vi "OP600ZP_Assembly.vi"(8 "DCIR_MESURES":cluster{dbl, dbl, dbl, dbl, dbl, dbl, dbl, dbl}) -> (0 "ToBDD":T1, 1 "Out":string, 3 "PASS/FAIL":bool)   [LabVIEW 2020]
uses:
  OP600ZP_VGConf.vi
  VG/PackType.vi
  VG/IS30%.vi
  VG/DCIR@1C.vi
  VG/Ubatt.vi
panel:
  out "errout":errorcluster caption="error out"
  in  "errin":errorcluster caption="error out"
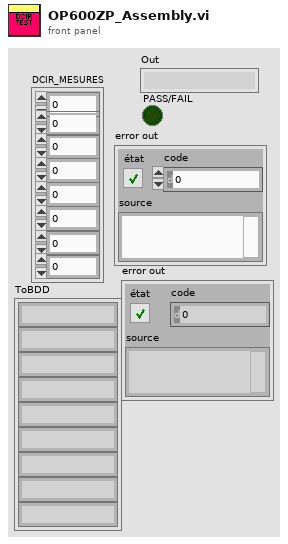
[diagram p1: front panel]
types:
  T1 = cluster{string, string, string, string, string, string, string, string, string}
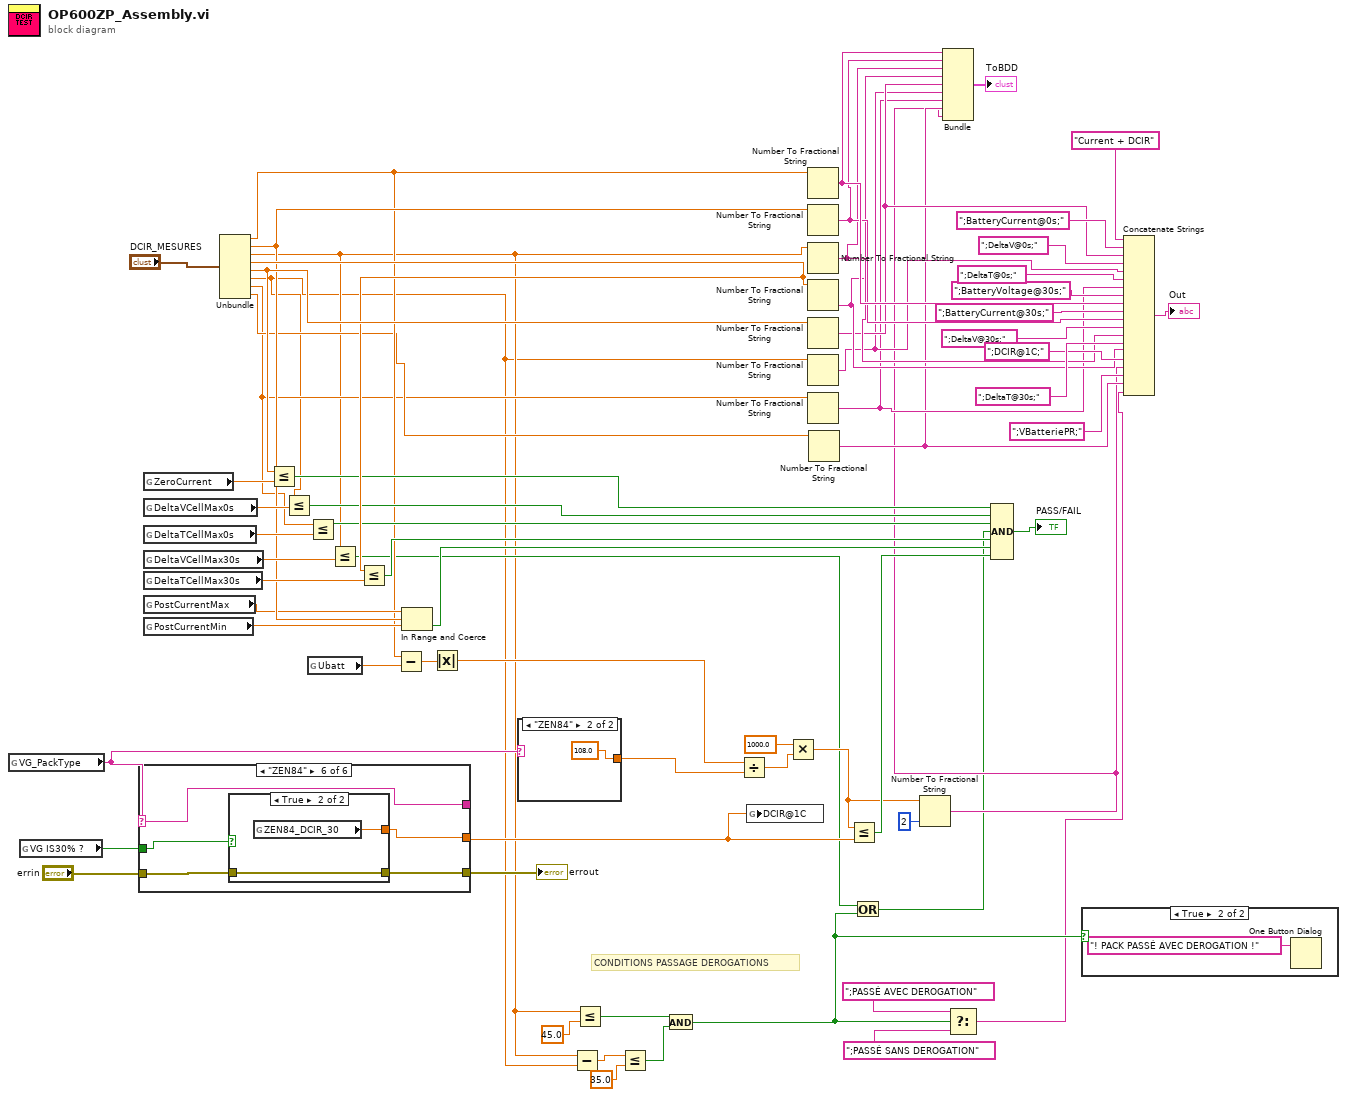
[diagram p0: block diagram]
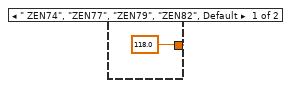
[diagram p3: hidden frame]
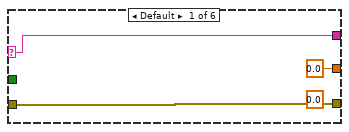
[diagram p4: hidden frame]
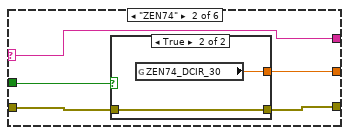
[diagram p5: hidden frame]
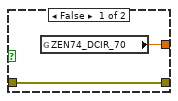
[diagram p6: hidden frame]
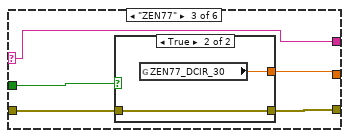
[diagram p7: hidden frame]
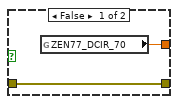
[diagram p8: hidden frame]
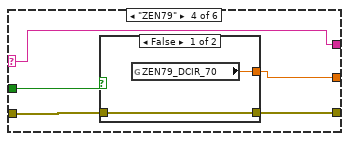
[diagram p9: hidden frame]
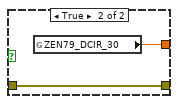
[diagram p10: hidden frame]
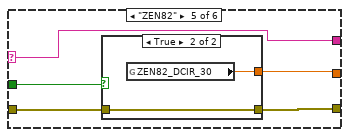
[diagram p11: hidden frame]
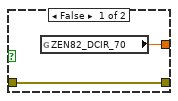
[diagram p12: hidden frame]
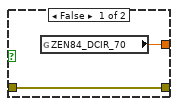
[diagram p13: hidden frame]
diagram:
  # "CONDITIONS PASSAGE DEROGATIONS"
  n1 = global read "PackType.vi" "VG_PackType"() -> (w36:string)
  n2 = global read "IS30%.vi" "VG IS30% ?"() -> (w42:bool)
  n3 = case shown="\"ZEN84\"" w36 {
    selector: w36 -> [w71 w74 w83 w92 w101 w110]
    tunnel: [0.0 ("ZEN84UbattMax30") w76 w85 w94 w103 w112] -> w32
    tunnel: w42 -> [_ w75 w84 w93 w102 w111]
    tunnel: [w71 w74 w83 w92 w101 w110] -> _
    tunnel: "errin" -> [w70 w73 w82 w91 w100 w109]
    tunnel: [w70 w72 w81 w90 w99 w108] -> w40
    frame Default {
      (unwired) 0.0 ("ZEN84UbattMin30")
    }
    frame "ZEN74" {
      n4 = case shown="True" w75 {
        tunnel: [w78 w80] -> w76
        tunnel: [w77 w79] -> w72
        tunnel: w73 -> [w77 w79]
        frame False {
          n5 = global read "OP600ZP_VGConf.vi" "ZEN74_DCIR_70"() -> (w78:dbl)
        }
        frame True {
          n6 = global read "OP600ZP_VGConf.vi" "ZEN74_DCIR_30"() -> (w80:dbl)
        }
      }
    }
    frame "ZEN77" {
      n7 = case shown="True" w84 {
        tunnel: [w87 w89] -> w85
        tunnel: w82 -> [w86 w88]
        tunnel: [w86 w88] -> w81
        frame False {
          n8 = global read "OP600ZP_VGConf.vi" "ZEN77_DCIR_70"() -> (w87:dbl)
        }
        frame True {
          n9 = global read "OP600ZP_VGConf.vi" "ZEN77_DCIR_30"() -> (w89:dbl)
        }
      }
    }
    frame "ZEN79" {
      n10 = case shown="False" w93 {
        tunnel: [w96 w98] -> w94
        tunnel: w91 -> [w95 w97]
        tunnel: [w95 w97] -> w90
        frame False {
          n11 = global read "OP600ZP_VGConf.vi" "ZEN79_DCIR_70"() -> (w96:dbl)
        }
        frame True {
          n12 = global read "OP600ZP_VGConf.vi" "ZEN79_DCIR_30"() -> (w98:dbl)
        }
      }
    }
    frame "ZEN82" {
      n13 = case shown="True" w102 {
        tunnel: [w105 w107] -> w103
        tunnel: w100 -> [w104 w106]
        tunnel: [w104 w106] -> w99
        frame False {
          n14 = global read "OP600ZP_VGConf.vi" "ZEN82_DCIR_70"() -> (w105:dbl)
        }
        frame True {
          n15 = global read "OP600ZP_VGConf.vi" "ZEN82_DCIR_30"() -> (w107:dbl)
        }
      }
    }
    frame "ZEN84" {
      n16 = case shown="True" w111 {
        tunnel: [w114 w116] -> w112
        tunnel: w109 -> [w113 w115]
        tunnel: [w113 w115] -> w108
        frame False {
          n17 = global read "OP600ZP_VGConf.vi" "ZEN84_DCIR_70"() -> (w114:dbl)
        }
        frame True {
          n18 = global read "OP600ZP_VGConf.vi" "ZEN84_DCIR_30"() -> (w116:dbl)
        }
      }
    }
  }
  "errout" <- w40
  n19 = global read "OP600ZP_VGConf.vi" "ZeroCurrent"() -> (w67:dbl)
  n20 = global read "OP600ZP_VGConf.vi" "DeltaVCellMax0s"() -> (w55:dbl)
  n21 = global read "OP600ZP_VGConf.vi" "DeltaTCellMax0s"() -> (w54:dbl)
  n22 = global read "OP600ZP_VGConf.vi" "DeltaVCellMax30s"() -> (w53:dbl)
  n23 = global read "OP600ZP_VGConf.vi" "DeltaTCellMax30s"() -> (w52:dbl)
  n24 = global read "OP600ZP_VGConf.vi" "PostCurrentMax"() -> (w49:dbl)
  n25 = global read "OP600ZP_VGConf.vi" "PostCurrentMin"() -> (w48:dbl)
  n26 = Unbundle("DCIR_MESURES") -> (w39:dbl, w50:dbl, w3:dbl, w51:dbl, w57:dbl, w2:dbl, w24:dbl, w26:dbl)
  n27 = Less Or Equal?(x=w57, y=w67) -> (x <= y?=w47:bool)
  n28 = Less Or Equal?(x=w2, y=w55) -> (x <= y?=w46:bool)
  n29 = Less Or Equal?(x=w24, y=w54) -> (x <= y?=w45:bool)
  n30 = global read "Ubatt.vi" "Ubatt"() -> (w38:dbl)
  n31 = Less Or Equal?(x=w3, y=w53) -> (x <= y?=w5:bool)
  n32 = Less Or Equal?(x=w51, y=w52) -> (x <= y?=w44:bool)
  n33 = Subtract(x=w39, y=w38) -> (x-y=w37:dbl)
  n34 = In Range and Coerce(upper limit=w49, x=w50, lower limit=w48) -> (In Range?=w43:bool)  [unwired: 1 out]
  n35 = Absolute Value(x=w37) -> (abs(x)=w35:dbl)
  n36 = case shown="\"ZEN84\"" w36 {
    tunnel: [118.0 108.0] -> w30
    frame " ZEN74", "ZEN77", "ZEN79", "ZEN82", Default {
    }
    frame "ZEN84" {
    }
  }
  n37 = Subtract(x=w3, y=w2) -> (x-y=w11:dbl)
  n38 = Less Or Equal?(x=w3, y=45.0) -> (x <= y?=w12:bool)
  n39 = Less Or Equal?(x=w11, y=35.0) -> (x <= y?=w9:bool)
  n40 = And(x=w12, y=w9) -> (x .and. y?=w6:bool)
  n41 = Divide(x=w35, y=w30) -> (x/y=w28:dbl)
  n42 = global write "DCIR@1C.vi" "DCIR@1C"(w32) -> ()
  n43 = Multiply(x=1000.0, y=w28) -> (x*y=w27:dbl)
  n44 = Number To Fractional String(number=w39) -> (F-format string=w23:string)  [unwired: 3 in]
  n45 = Number To Fractional String(number=w50) -> (F-format string=w22:string)  [unwired: 3 in]
  n46 = Number To Fractional String(number=w3) -> (F-format string=w21:string)  [unwired: 3 in]
  n47 = Number To Fractional String(number=w51) -> (F-format string=w20:string)  [unwired: 3 in]
  n48 = Number To Fractional String(number=w57) -> (F-format string=w19:string)  [unwired: 3 in]
  n49 = Number To Fractional String(number=w2) -> (F-format string=w18:string)  [unwired: 3 in]
  n50 = Number To Fractional String(number=w24) -> (F-format string=w17:string)  [unwired: 3 in]
  n51 = Number To Fractional String(number=w26) -> (F-format string=w16:string)  [unwired: 3 in]
  n52 = Less Or Equal?(x=w27, y=w32) -> (x <= y?=w31:bool)
  n53 = Or(x=w5, y=w6) -> (x .or. y?=w4:bool)
  n54 = Number To Fractional String(number=w27, precision (6)=i16 2 ("précision (6)")) -> (F-format string=w15:string)  [unwired: 2 in]
  n55 = Bundle(w23, w22, w21, w20, w19, w18, w17, w16, w15) -> (→"ToBDD":T1)  [unwired: 1 in]
  n56 = Select(t=";PASSÉ AVEC DEROGATION", s=w6, f=";PASSÉ SANS DEROGATION") -> (s? t:f=w1:string)
  n57 = Compound Arithmetic op=AND ("Opérateur arithmétique")(w47, w46, w45, w4, w44, w43, w31) -> (→"PASS/FAIL":bool)
  n58 = case shown="True" w6 {
    frame False {
    }
    frame True {
      n59 = One Button Dialog(message="! PACK PASSÉ AVEC DEROGATION !") -> ()  [unwired: 1 in, 1 out]
    }
  }
  n60 = Concatenate Strings("Current + DCIR" ("élément"), ";BatteryCurrent@0s;" ("élément"), w19, ";DeltaV@0s;" ("élément"), w18, ";DeltaT@0s;" ("élément"), w17, ";BatteryVoltage@30s;" ("élément"), w23, ";BatteryCurrent@30s;" ("élément"), w22, ";DeltaV@30s;" ("élément"), w21, ";DeltaT@30s;" ("élément"), w20, ";DCIR@1C;" ("chaîne"), w15, ";VBatteriePR;" ("chaîne"), w16, w1) -> (→"Out":string)
